vi "BuildCall.vi"(7 "PythonConverter_BD in":refnum<class "PyConvBD.lvclass">, 8 "error in":errorcluster, 11 "Function in":refnum<class "Function.lvclass">) -> (0 "error out":errorcluster, 3 "Function out":refnum<class "Function.lvclass">, 5 "PythonConverter_BD out":refnum<class "PyConvBD.lvclass">)   [LabVIEW 2014, in "Function.lvclass"]
uses:
  Function.lvclass
  Python/PythonConverter_BD/PyConvBD.lvclass
  Python/Parsing/Classes/PythonFunction/PythonFunction.lvclass/PythonFunction.ctl
  Python/PythonConverter_BD/TypeDefs/NodeCall_TD.ctl
  Python/Parsing/ListTypesTD.ctl
  Python/Parsing/Classes/PythonFunction/PythonFunction.lvclass
  Python/Parsing/Python Functions.lvlib
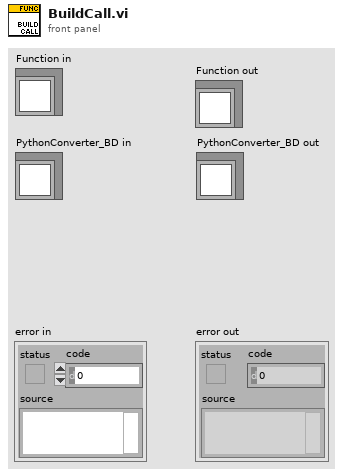
[diagram p1: front panel]
types:
  T1 = typedef "Python Functions.lvlib/ListTypesTD.ctl" = enum16{"list", "tuple", "parameter list", "output list"}
  T2 = typedef "NodeCall_TD.ctl" = cluster{"call":string, "collect":string, "Threaded":bool, "branches":string[]}
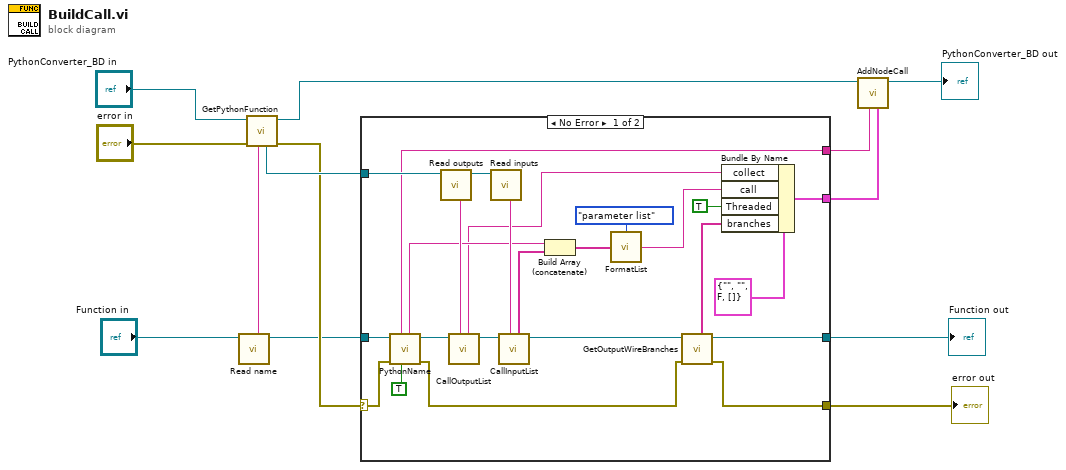
[diagram p0: block diagram]
diagram:
  n1 = call-dynamic "Read name.vi"("Node in"="Function in") -> ("Node out"=w7:refnum<class "Function.lvclass">, "name"=w8:string)  [unwired: 7 in]
  n2 = call "GetPythonFunction.vi"("function name"=w8, "error in"="error in", "PythonConverter_BD in"="PythonConverter_BD in") -> ("error out"=w12:errorcluster, "PythonConverter_BD out"=w11:refnum<class "PyConvBD.lvclass">, "Python function"=w13:refnum<class "PythonFunction.lvclass">)  [unwired: 4 in]
  n3 = case shown="No Error" w12 {
    selector: w12 -> [w33 w39]
    tunnel: [w15 w39] -> w4
    tunnel: [w23 _] -> w10
    tunnel: w7 -> [w32 w38]
    tunnel: w13 -> [w35 _]
    tunnel: [w31 _] -> w9
    tunnel: [w17 w38] -> w5
    frame No Error {
      n4 = call-dynamic "PythonName.vi"("add self"=TRUE, "error in"=w33, "Node in"=w32) -> ("error out"=w16:errorcluster, "Node out"=w28:refnum<class "Function.lvclass">, "name"=w30:string, "UID"=w31:string)  [unwired: 5 in]
      n5 = call "Read outputs.vi"("PythonFunction in"=w35) -> ("PythonFunction out"=w34:refnum<class "PythonFunction.lvclass">, "outputs"=w37:string)  [unwired: 7 in]
      n6 = call-dynamic "CallOutputList.vi"("list"=w37, "Function in"=w28) -> ("Function out"=w27:refnum<class "Function.lvclass">, "call outputs"=w20:string)  [unwired: 6 in]
      n7 = call "Read inputs.vi"("PythonFunction in"=w34) -> ("inputs"=w36:string)  [unwired: 7 in, 1 out]
      n8 = call-dynamic "CallInputList.vi"("list"=w36, "Function in"=w27) -> ("Function out"=w18:refnum<class "Function.lvclass">, "call inputs"=w29:string[])  [unwired: 6 in]
      n9 = Build Array (concatenate)(w30, w29) -> (w21:string[])
      n10 = call "FormatList.vi"("values"=w21, "type"=ListTypesTD."parameter list") -> ("python object"=w19:string)
      n11 = call-dynamic "GetOutputWireBranches.vi"("error in"=w16, "Node in"=w18) -> ("error out"=w15:errorcluster, "Node out"=w17:refnum<class "Function.lvclass">, "branches"=w14:string[])  [unwired: 5 in]
      n12 = Bundle By Name(cluster=T2 {"call"="", "collect"="", "Threaded"=FALSE, "branches"=[]} ("call"), "collect"=w20, "call"=w19, "Threaded"=TRUE, "branches"=w14) -> (w23:T2)
    }
    frame Error {
    }
  }
  "error out" <- w4
  "Function out" <- w5
  n13 = call "AddNodeCall.vi"("call"=w10, "name"=w9, "PythonConverter_BD in"=w11) -> ("PythonConverter_BD out"=→"PythonConverter_BD out":refnum<class "PyConvBD.lvclass">)  [unwired: 5 in, 1 out]
